vi "sshExec.vi"(8 "error in":errorcluster, 10 "Commands":string[](array[string]), 11 "ConnectionData":T1) -> (0 "error out":errorcluster, 3 "Output":string[](array[string]))   [LabVIEW 2015]
uses:
  connectionData.ctl
panel:
  # "Executes remote commands on the target device via SSH, using the plink utility. \nThis VI expects to find plink.exe in the same dirctory that this VI is located in.\nDOWNLOAD: http://www.chiark.greenend.org.uk/~sgtatham/putty/download.html"
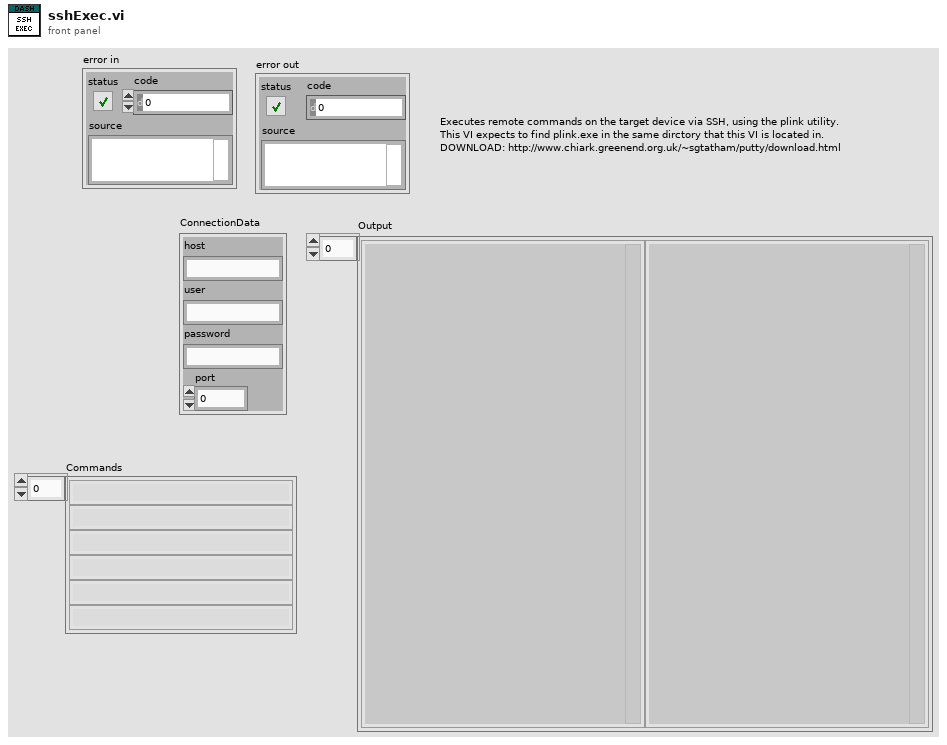
[diagram p1: front panel]
types:
  T1 = typedef "connectionData.ctl" = cluster{"host":string, "user":string, "password":string, "port":u16}
  T2 = enum16{"open", "replace", "create", "open or create", "replace or create", "replace or create with confirmation"}
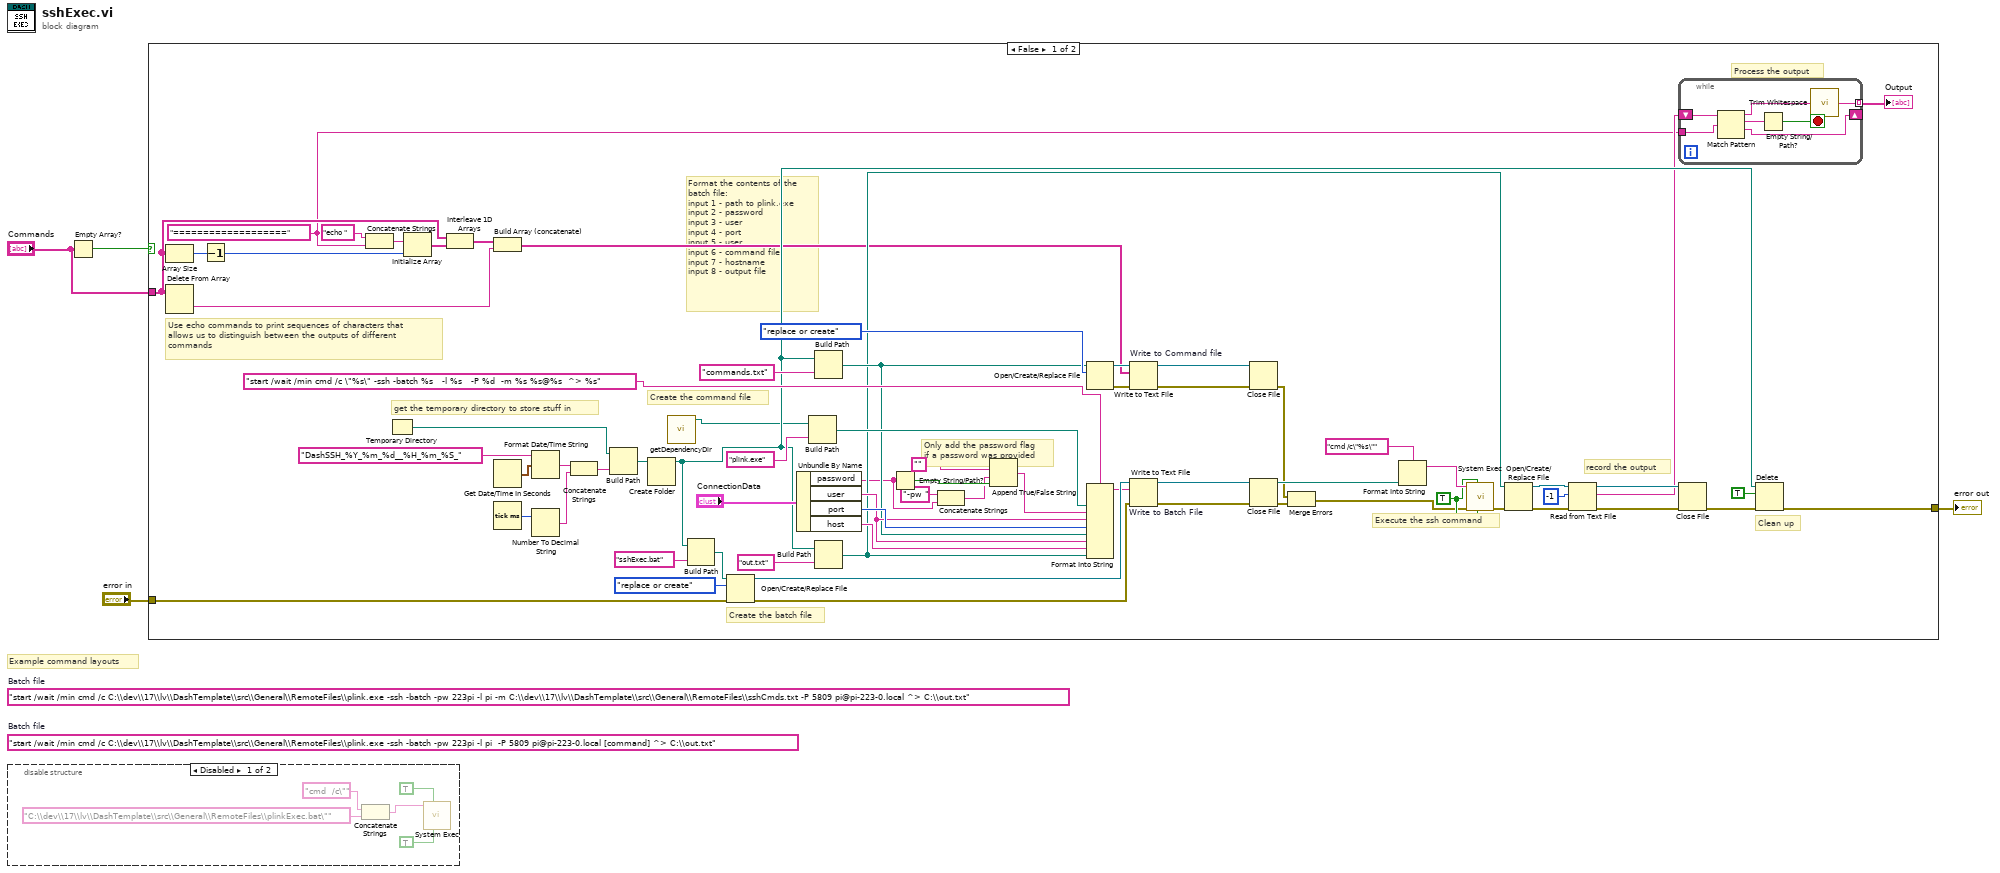
[diagram p0: block diagram]
diagram:
  (unwired) "start /wait /min cmd /c C:\\dev\\17\\lv\\DashTemplate\\src\\General\\RemoteFiles\\plink.exe -ssh -batch -pw 223pi -l pi  -P 5809 pi@pi-223-0.local [command] ^> C:\\out.txt"  # Batch file
  (unwired) "start /wait /min cmd /c C:\\dev\\17\\lv\\DashTemplate\\src\\General\\RemoteFiles\\plink.exe -ssh -batch -pw 223pi -l pi -m C:\\dev\\17\\lv\\DashTemplate\\src\\General\\RemoteFiles\\sshCmds.txt -P 5809 pi@pi-223-0.local ^> C:\\out.txt"  # Batch file
  # "Example command layouts"
  n1 = disable-structure shown="Disabled" {
    frame Disabled {
      n2 = Concatenate Strings("cmd  /c\"" ("command line"), "C:\\dev\\17\\lv\\DashTemplate\\src\\General\\RemoteFiles\\plinkExec.bat\"" ("standard input")) -> (w5:string)
      n3 = call <vilib>:"System Exec.vi"("run minimized? (F)"=TRUE, "wait until completion? (T)"=TRUE, "command line"=w5) -> ()  [unwired: 5 in, 4 out]
    }
    frame Enabled {
    }
  }
  n4 = Empty Array?(array="Commands") -> (empty?=w2:bool)
  n5 = case shown="False" w2 {
    tunnel: "Commands" -> [w24 _]
    tunnel: [w30 w86] -> w4
    tunnel: "error in" -> [w31 w86]
    frame False {
      w18 = "===================" ("string")
      w44 = TRUE ("wait until completion? (T)")
      # "Clean up"
      # "Only add the password flag\nif a password was provided"
      # "Process the output"
      # "Use echo commands to print sequences of characters that\nallows us to distinguish between the outputs of different\ncommands"
      # "record the output"
      # "Execute the ssh command"
      # "Create the batch file"
      # "Create the command file"
      # "get the temporary directory to store stuff in"
      # "Format the contents of the \nbatch file:\ninput 1 - path to plink.exe\ninput 2 - password\ninput 3 - user\ninput 4 - port\ninput 5 - user\ninput 6 - command file\ninput 7 - hostname\ninput 8 - output file"
      n6 = Array Size(array=w24) -> (size(s)=w29:i32)
      n7 = Delete From Array(array=w24) -> (deleted portion=w25:string)  [unwired: 2 in, 1 out]
      n8 = Decrement(x=w29) -> (x-1=w28:i32)
      n9 = Concatenate Strings("echo " ("decimal integer string"), w18) -> (w21:string)
      n10 = Temporary Directory() -> (w72:path)
      n11 = Initialize Array(w21, w28) -> (w27:string[])
      n12 = Interleave 1D Arrays(w24, w27) -> (w26:string[])
      n13 = Build Array (concatenate)(w26, w25) -> (w23:string[])
      n14 = Get Date/Time In Seconds() -> (seconds since 1Jan1904=w71:timestamp)
      n15 = Tick Count (ms)() -> (millisecond timer value=w67:u32)
      n16 = Format Date/Time String(time format string (%c)="DashSSH_%Y_%m_%d__%H_%m_%S_", seconds (now)=w71) -> (date/time string=w69:string)  [unwired: 1 in]
      n17 = Number To Decimal String(number=w67) -> (decimal integer string=w66:string)  [unwired: 1 in]
      n18 = Concatenate Strings(w69, w66) -> (w68:string)
      n19 = Build Path(base path=w72, name or relative path=w68) -> (appended path=w65:path)
      n20 = Create Folder(path (use dialog)=w65) -> (created path=w38:path)  [unwired: 2 in, 2 out]
      n21 = call "getDependencyDir.vi"() -> ("Dependency Directory"=w11:path)  [unwired: 11 in]
      n22 = Build Path(base path=w38, name or relative path="sshExec.bat") -> (appended path=w60:path)
      n23 = Open/Create/Replace File(file path (use dialog)=w60, error in=w31, operation (0:open)=T2."replace or create") -> (refnum out=w58:refnum<file>, error out=w57:errorcluster)  [unwired: 3 in, 1 out]
      n24 = Unbundle By Name("ConnectionData") -> ("password"=w13:string, "user"=w62:string, "port"=w74:u16, "host"=w73:string)
      n25 = Build Path(base path=w11, name or relative path="plink.exe") -> (appended path=w76:path)
      n26 = Build Path(base path=w38, name or relative path="commands.txt") -> (appended path=w48:path)
      n27 = Build Path(base path=w38, name or relative path="out.txt") -> (appended path=w42:path)
      n28 = Empty String/Path?(string/path=w13) -> (empty?=w17:bool)
      n29 = Concatenate Strings("-pw " ("string"), w13) -> (w14:string)
      n30 = Append True/False String(1:w17, 2:w14, 3:"") -> (0:w12:string)  [unwired: 1 in]
      n31 = Open/Create/Replace File(file path (use dialog)=w48, operation (0:open)=T2."replace or create") -> (refnum out=w50:refnum<file>, error out=w51:errorcluster)  [unwired: 4 in, 1 out]
      n32 = Format Into String(format string="start /wait /min cmd /c \"%s\" -ssh -batch %s   -l %s   -P %d  -m %s %s@%s  ^> %s", w76, w12, w62, w74, w48, w62, w73, w42) -> (resulting string=w56:string)  [unwired: 2 in, 1 out]
      n33 = Write to Text File "Write to Command file"(file (use dialog)=w50, text=w23, error in=w51) -> (refnum out=w53:refnum<file>, error out=w52:errorcluster)  [unwired: 1 in, 1 out]
      n34 = Write to Text File "Write to Batch File"(file (use dialog)=w58, text=w56, error in=w57) -> (refnum out=w54:refnum<file>, error out=w55:errorcluster)  [unwired: 1 in, 1 out]
      n35 = Close File(refnum=w53, error in=w52) -> (error out=w36:errorcluster)  [unwired: 1 out]
      n36 = Close File(refnum=w54, error in=w55) -> (path=w46:path, error out=w37:errorcluster)
      n37 = Merge Errors(w36, w37) -> (w35:errorcluster)
      n38 = Format Into String(format string="cmd /c\"%s\"", w46) -> (resulting string=w45:string)  [unwired: 2 in, 1 out]
      n39 = call <vilib>:"System Exec.vi"("run minimized? (F)"=w44, "wait until completion? (T)"=w44, "error in (no error)"=w35, "command line"=w45) -> ("error out"=w43:errorcluster)  [unwired: 4 in, 3 out]
      n40 = Open/Create/Replace File(file path (use dialog)=w42, error in=w43) -> (refnum out=w40:refnum<file>, error out=w41:errorcluster)  [unwired: 4 in, 1 out]
      n41 = Read from Text File(file (use dialog)=w40, count=-1, error in=w41) -> (refnum out=w34:refnum<file>, text=w20:string, error out=w33:errorcluster)  [unwired: 1 in, 1 out]
      n42 = while {
        shift-right: [w83] -> _
        shift-left: w20 -> [w85]
        tunnel: w18 -> [w84]
        tunnel: [w79] -> w19 mode=indexing
        stop <- w81 stop-if-true
        n43 = Match Pattern(string=w85, regular expression=w84) -> (before substring=w80:string, match substring=w82:string, after substring=w83:string)  [unwired: 1 in, 1 out]
        n44 = Empty String/Path?(string/path=w82) -> (empty?=w81:bool)
        n45 = call <vilib>:"Trim Whitespace.vi"("string"=w80) -> ("trimmed string"=w79:string)  [unwired: 1 in]
      }
      "Output" <- w19
      n46 = Close File(refnum=w34, error in=w33) -> (error out=w32:errorcluster)  [unwired: 1 out]
      n47 = Delete(path (use dialog)=w38, entire hierarchy (F)=TRUE, error in=w32) -> (error out=w30:errorcluster)  [unwired: 2 in, 2 out]
    }
    frame True {
      # "Only run if commands have been supplied, or else plink will hang"
    }
  }
  "error out" <- w4
